vi "GFITS_processOneExt.vi"(6 "def_timing":string="after", 9 "starting line":u16, 10 "line string":string, 11 "config file":path) -> (1 "finished":bool, 2 "number of keywords":i32, 3 "Extension Keywords":string[][](table), 5 "number of before keywords":i32, 7 "Extension before keywords":string[][](array[string]))   [LabVIEW 2016]
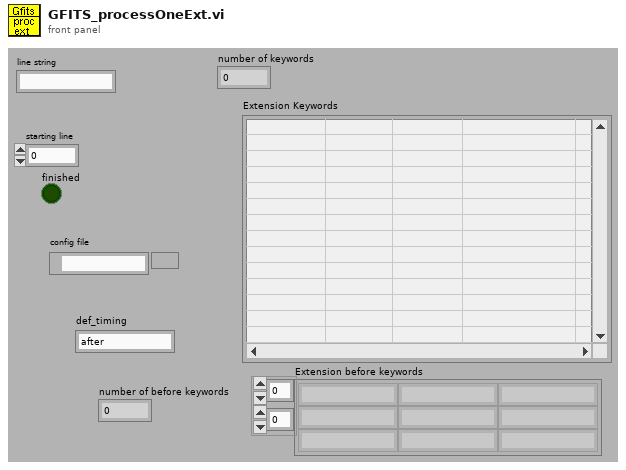
[diagram p1: front panel]
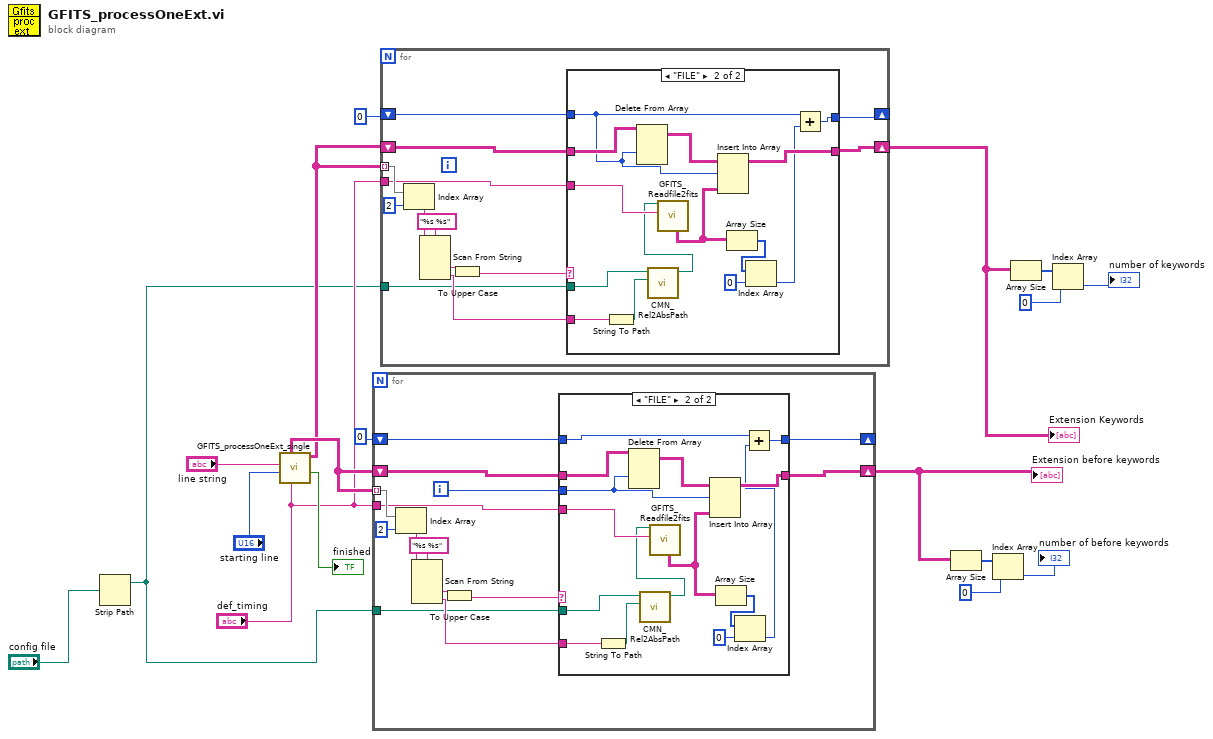
[diagram p0: block diagram]
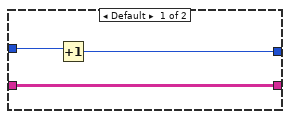
[diagram p2: hidden frame]
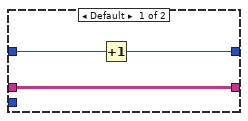
[diagram p3: hidden frame]
diagram:
  n1 = Strip Path(path="config file") -> (stripped path=w3:path)  [unwired: 1 out]
  n2 = call "GFITS_processOneExt_single.vi"("def_timing"="def_timing", "starting line"="starting line", "line string"="line string") -> ("finished"=→"finished":bool, "Extension Keywords"=w10:string[][], "Extension before keywords"=w16:string[][])  [unwired: 6 out]
  n3 = for {
    shift-right: [w25] -> w15
    shift-left: w16 -> [w26]
    tunnel: w16 -> [w32] mode=indexing
    tunnel: "def_timing" -> [w24]
    tunnel: w3 -> [w21]
    shift-right: [w19] -> _
    shift-left: 0 -> [w20]
    i -> [w23]
    n4 = Index Array(array=w32, index=2) -> (element=w30:string)
    n5 = Scan From String(format string="%s %s", input string=w30) -> (output 1=w28:string, output 2=w22:string)  [unwired: 2 in, 5 out]
    n6 = To Upper Case(1:w28) -> (0:w27:string)
    n7 = case shown="\"FILE\"" w27 {
      tunnel: w26 -> [w35 w45]
      tunnel: [w35 w49] -> w25
      tunnel: w24 -> [_ w50]
      tunnel: w23 -> [_ w44]
      tunnel: w22 -> [_ w46]
      tunnel: w21 -> [_ w42]
      tunnel: w20 -> [w34 w37]
      tunnel: [w33 w36] -> w19
      frame Default {
        n8 = Increment(x=w34) -> (x+1=w33:i32)
      }
      frame "FILE" {
        n9 = String To Path(string=w46) -> (path=w48:path)
        n10 = Delete From Array(array=w45, index (row)=w44) -> (array with subset deleted=w43:string[][])  [unwired: 2 in, 1 out]
        n11 = call "CMN_Rel2AbsPath.vi"("test path"=w48, "absolute path"=w42) -> ("output path"=w47:path)  [unwired: 1 in, 8 out]
        n12 = call "GFITS_Readfile2fits.vi"("def_timing"=w50, "file"=w47) -> ("all keys"=w39:string[][])  [unwired: 9 out]
        n13 = Insert Into Array(array=w43, index (row)=w44, new element=w39) -> (w49:string[][])  [unwired: 1 in]
        n14 = Array Size(array=w39) -> (size(s)=w41:i32[])
        n15 = Index Array(array=w41, index=0) -> (element=w38:i32)
        n16 = Add(x=w37, y=w38) -> (x+y=w36:i32)
      }
    }
  }
  "Extension before keywords" <- w15
  n17 = for {
    shift-right: [w56] -> w6
    shift-left: w10 -> [w57]
    tunnel: w10 -> [w63] mode=indexing
    tunnel: "def_timing" -> [w55]
    tunnel: w3 -> [w53]
    shift-right: [w51] -> _
    shift-left: 0 -> [w52]
    n18 = Index Array(array=w63, index=2) -> (element=w61:string)
    n19 = Scan From String(format string="%s %s", input string=w61) -> (output 1=w59:string, output 2=w54:string)  [unwired: 2 in, 5 out]
    n20 = To Upper Case(1:w59) -> (0:w58:string)
    n21 = case shown="\"FILE\"" w58 {
      tunnel: w57 -> [w66 w75]
      tunnel: [w66 w79] -> w56
      tunnel: w55 -> [_ w80]
      tunnel: w54 -> [_ w76]
      tunnel: w53 -> [_ w73]
      tunnel: w52 -> [w65 w67]
      tunnel: [w64 w68] -> w51
      frame Default {
        n22 = Increment(x=w65) -> (x+1=w64:i32)
      }
      frame "FILE" {
        n23 = String To Path(string=w76) -> (path=w78:path)
        n24 = Delete From Array(array=w75, index (row)=w67) -> (array with subset deleted=w74:string[][])  [unwired: 2 in, 1 out]
        n25 = call "CMN_Rel2AbsPath.vi"("test path"=w78, "absolute path"=w73) -> ("output path"=w77:path)  [unwired: 1 in, 8 out]
        n26 = call "GFITS_Readfile2fits.vi"("def_timing"=w80, "file"=w77) -> ("all keys"=w72:string[][])  [unwired: 9 out]
        n27 = Insert Into Array(array=w74, index (row)=w67, new element=w72) -> (w79:string[][])  [unwired: 1 in]
        n28 = Array Size(array=w72) -> (size(s)=w71:i32[])
        n29 = Index Array(array=w71, index=0) -> (element=w69:i32)
        n30 = Add(x=w67, y=w69) -> (x+y=w68:i32)
      }
    }
  }
  "Extension Keywords" <- w6
  n31 = Array Size(array=w15) -> (size(s)=w14:i32[])
  n32 = Index Array(array=w14, index=0) -> (element=→"number of before keywords":i32)
  n33 = Array Size(array=w6) -> (size(s)=w8:i32[])
  n34 = Index Array(array=w8, index=0) -> (element=→"number of keywords":i32)
